vi "水样测试.vi"(11 "数据标记表":string(combo)="N") -> ()   [LabVIEW 2016, in "斯坦道多参数.lvlib"]
panel:
  out "运行状态":u16(ring) items=["空闲", "水样测试", "标样核查"]
  out "多参数运行日志":string
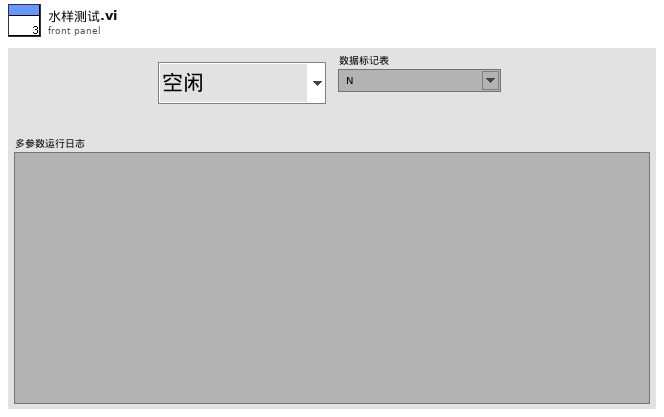
[diagram p1: front panel]
types:
  T1 = cluster{"因子编码":string, "单位":string, "标样参考值":sgl, "水样数据时间":timestamp, "水样实测值":sgl, "水样数据标识":string, "探头温度":sgl}
  T2 = cluster{"温度测量值":sgl, "DO%":sgl, "DOmg/L":sgl, "温度偏移修正值":sgl}
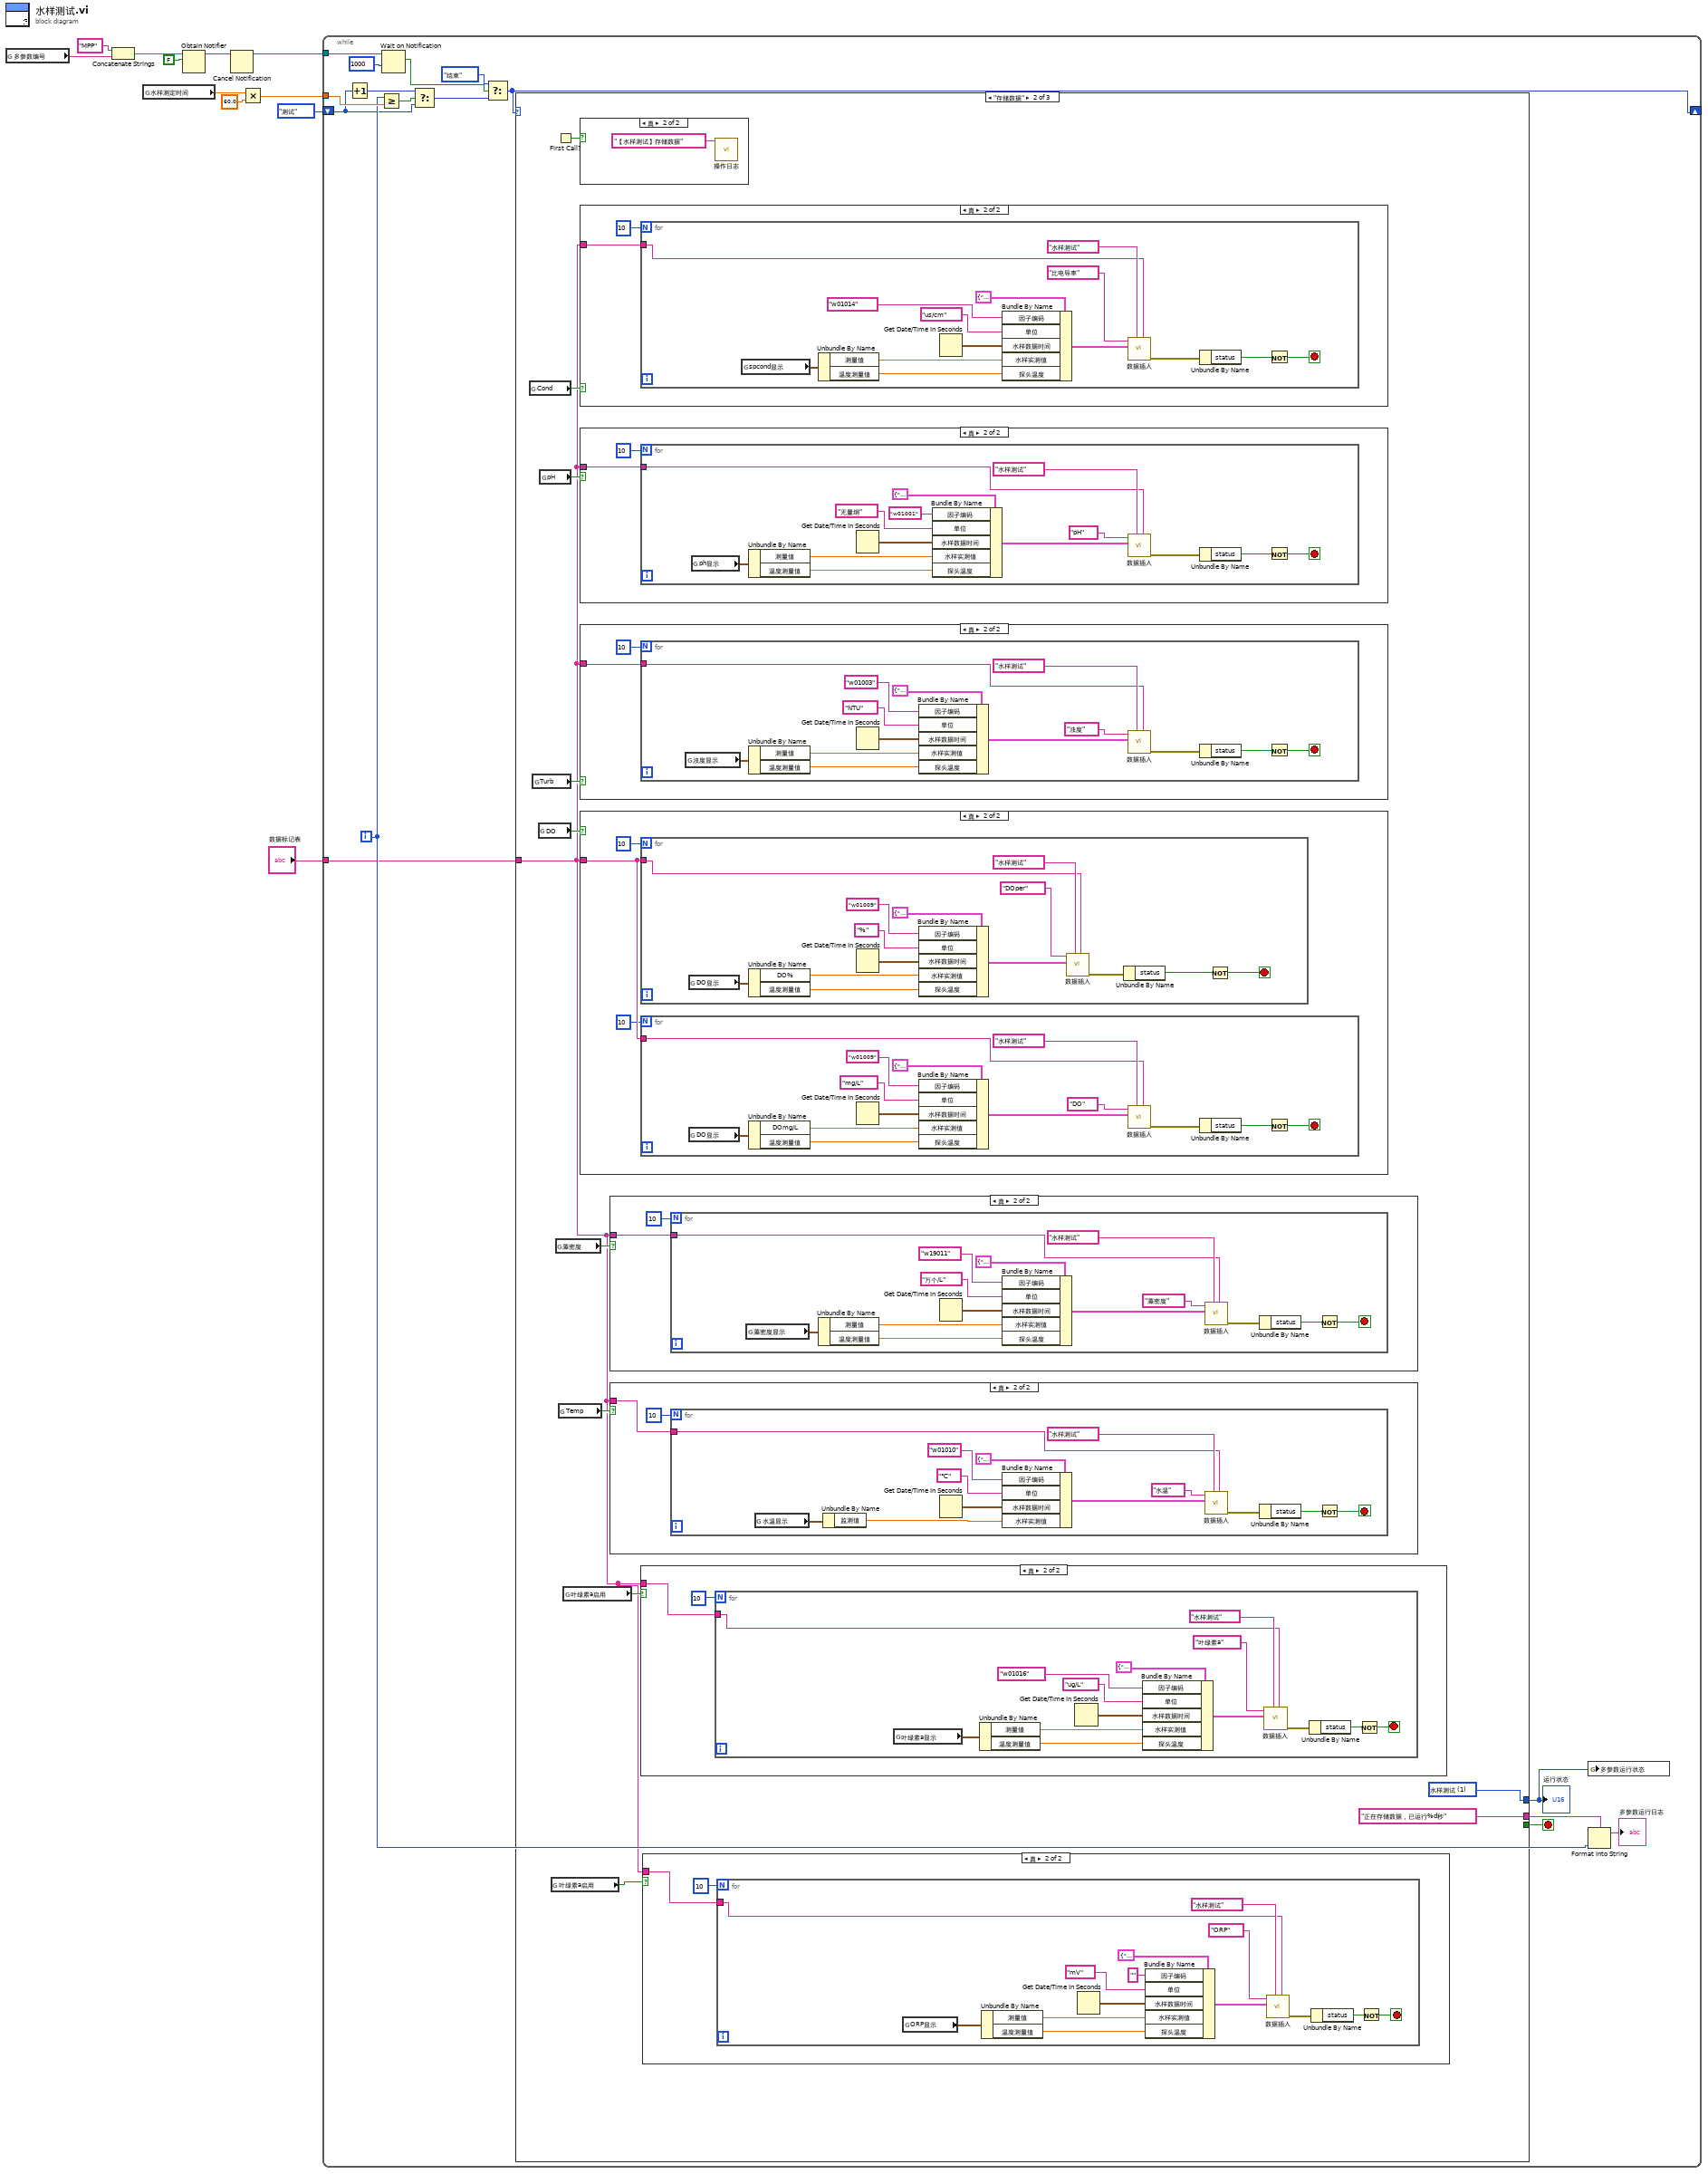
[diagram p0: block diagram]
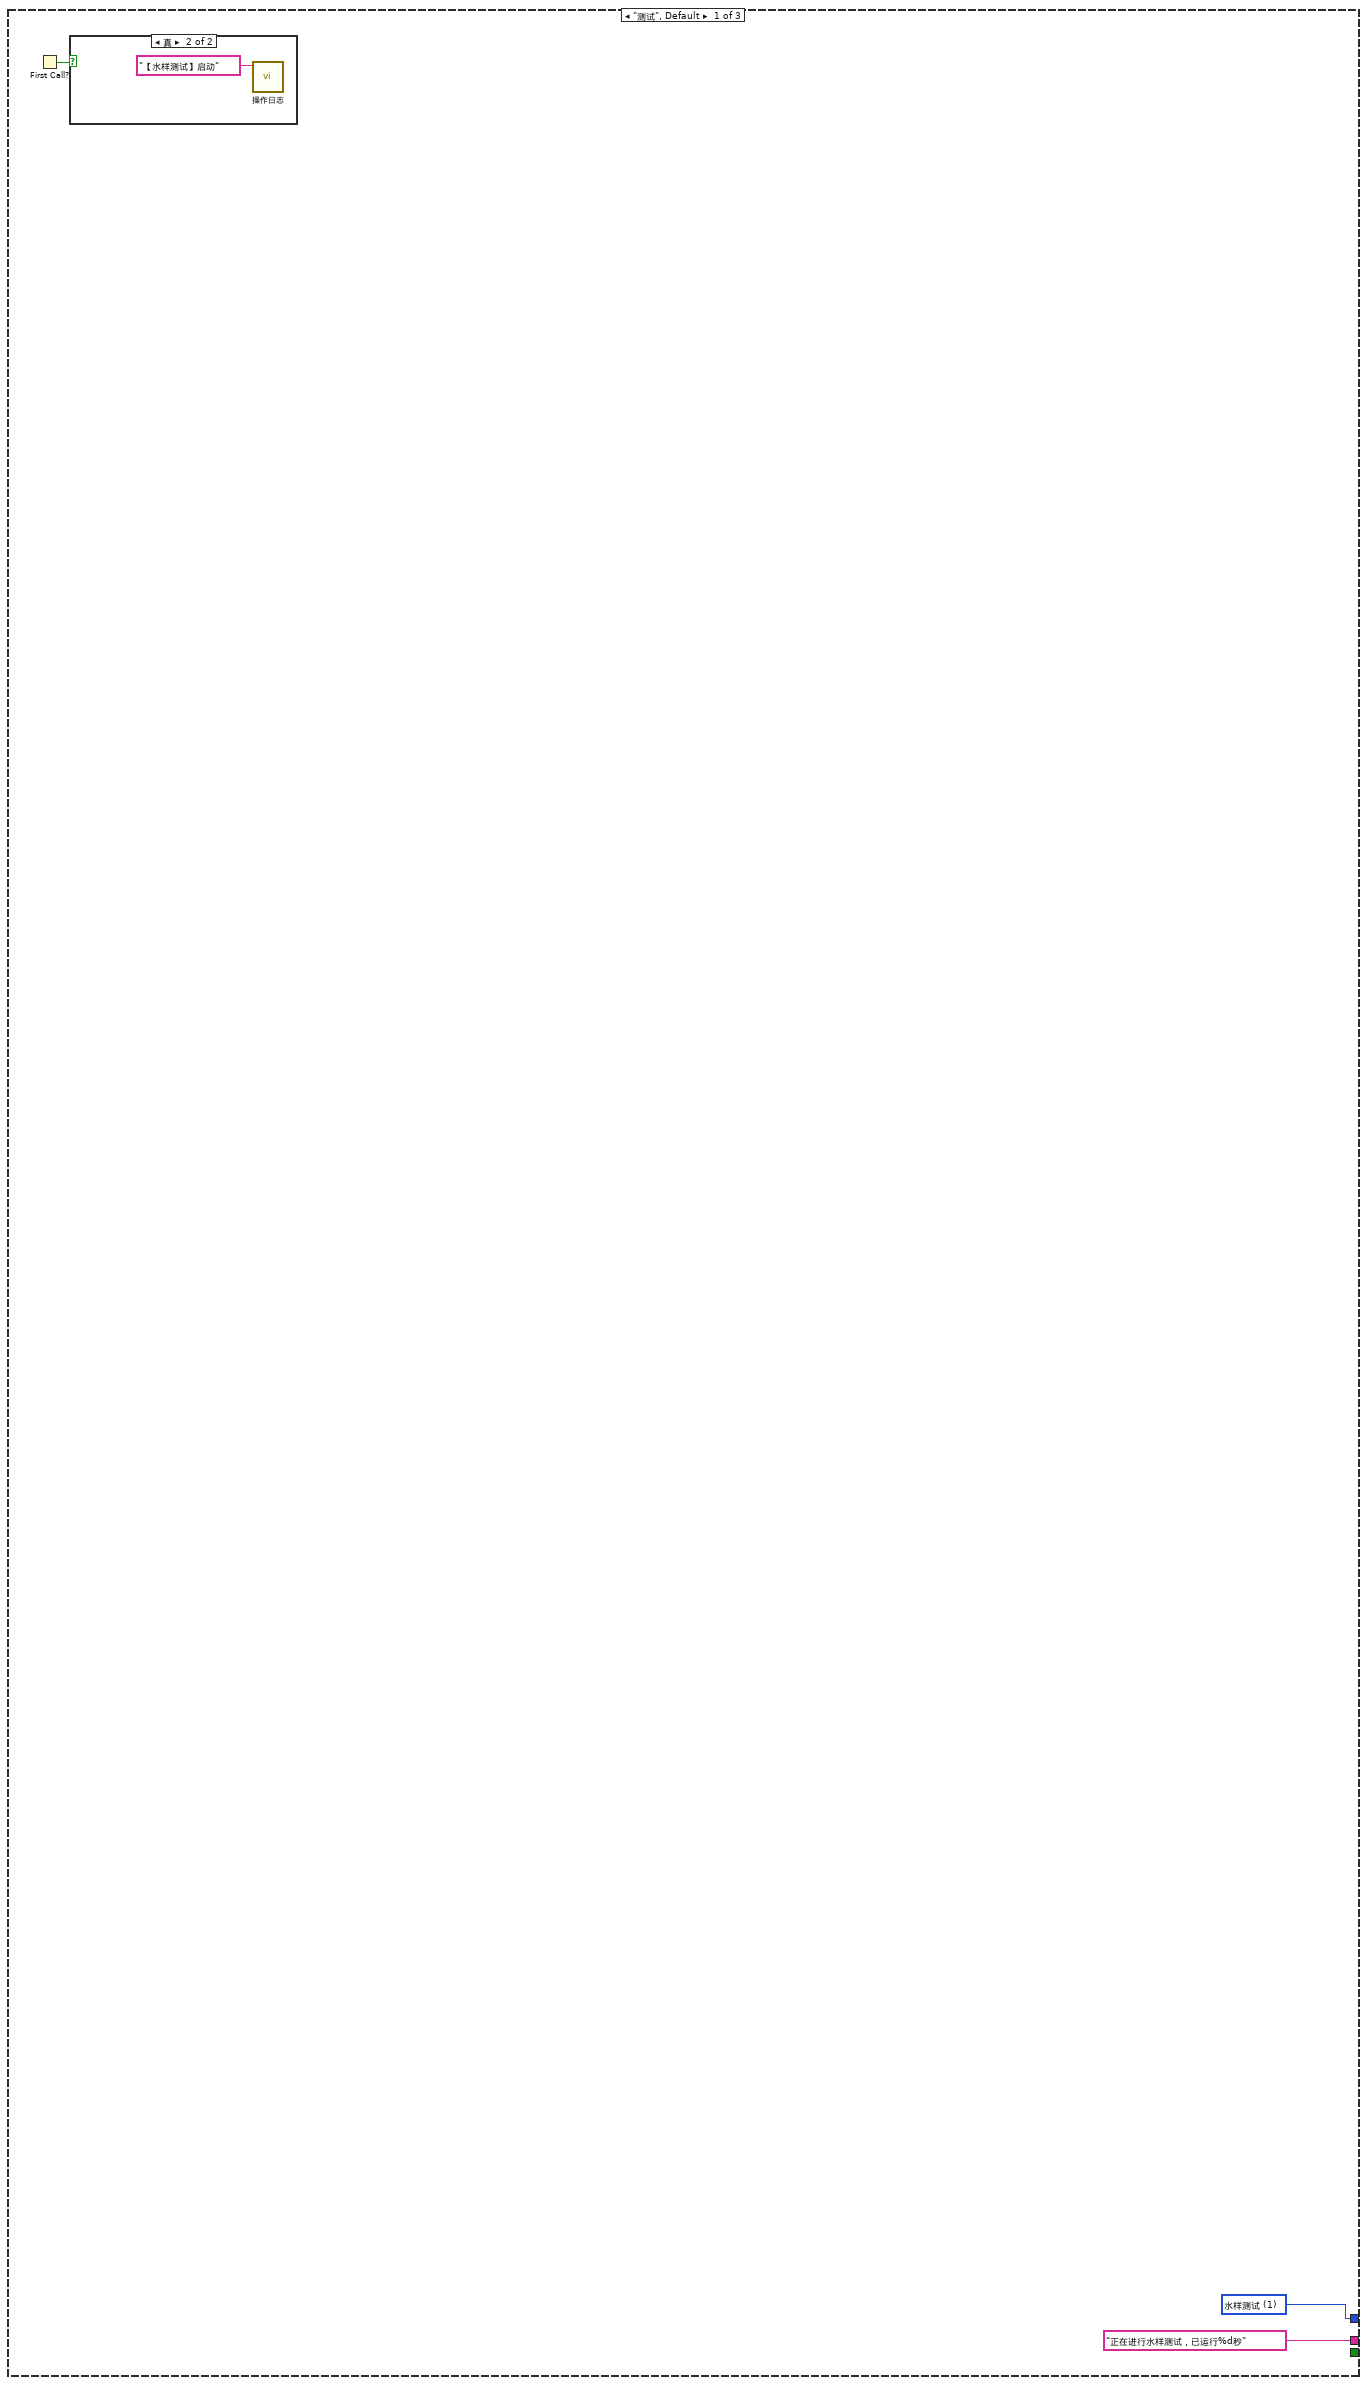
[diagram p2: hidden frame]
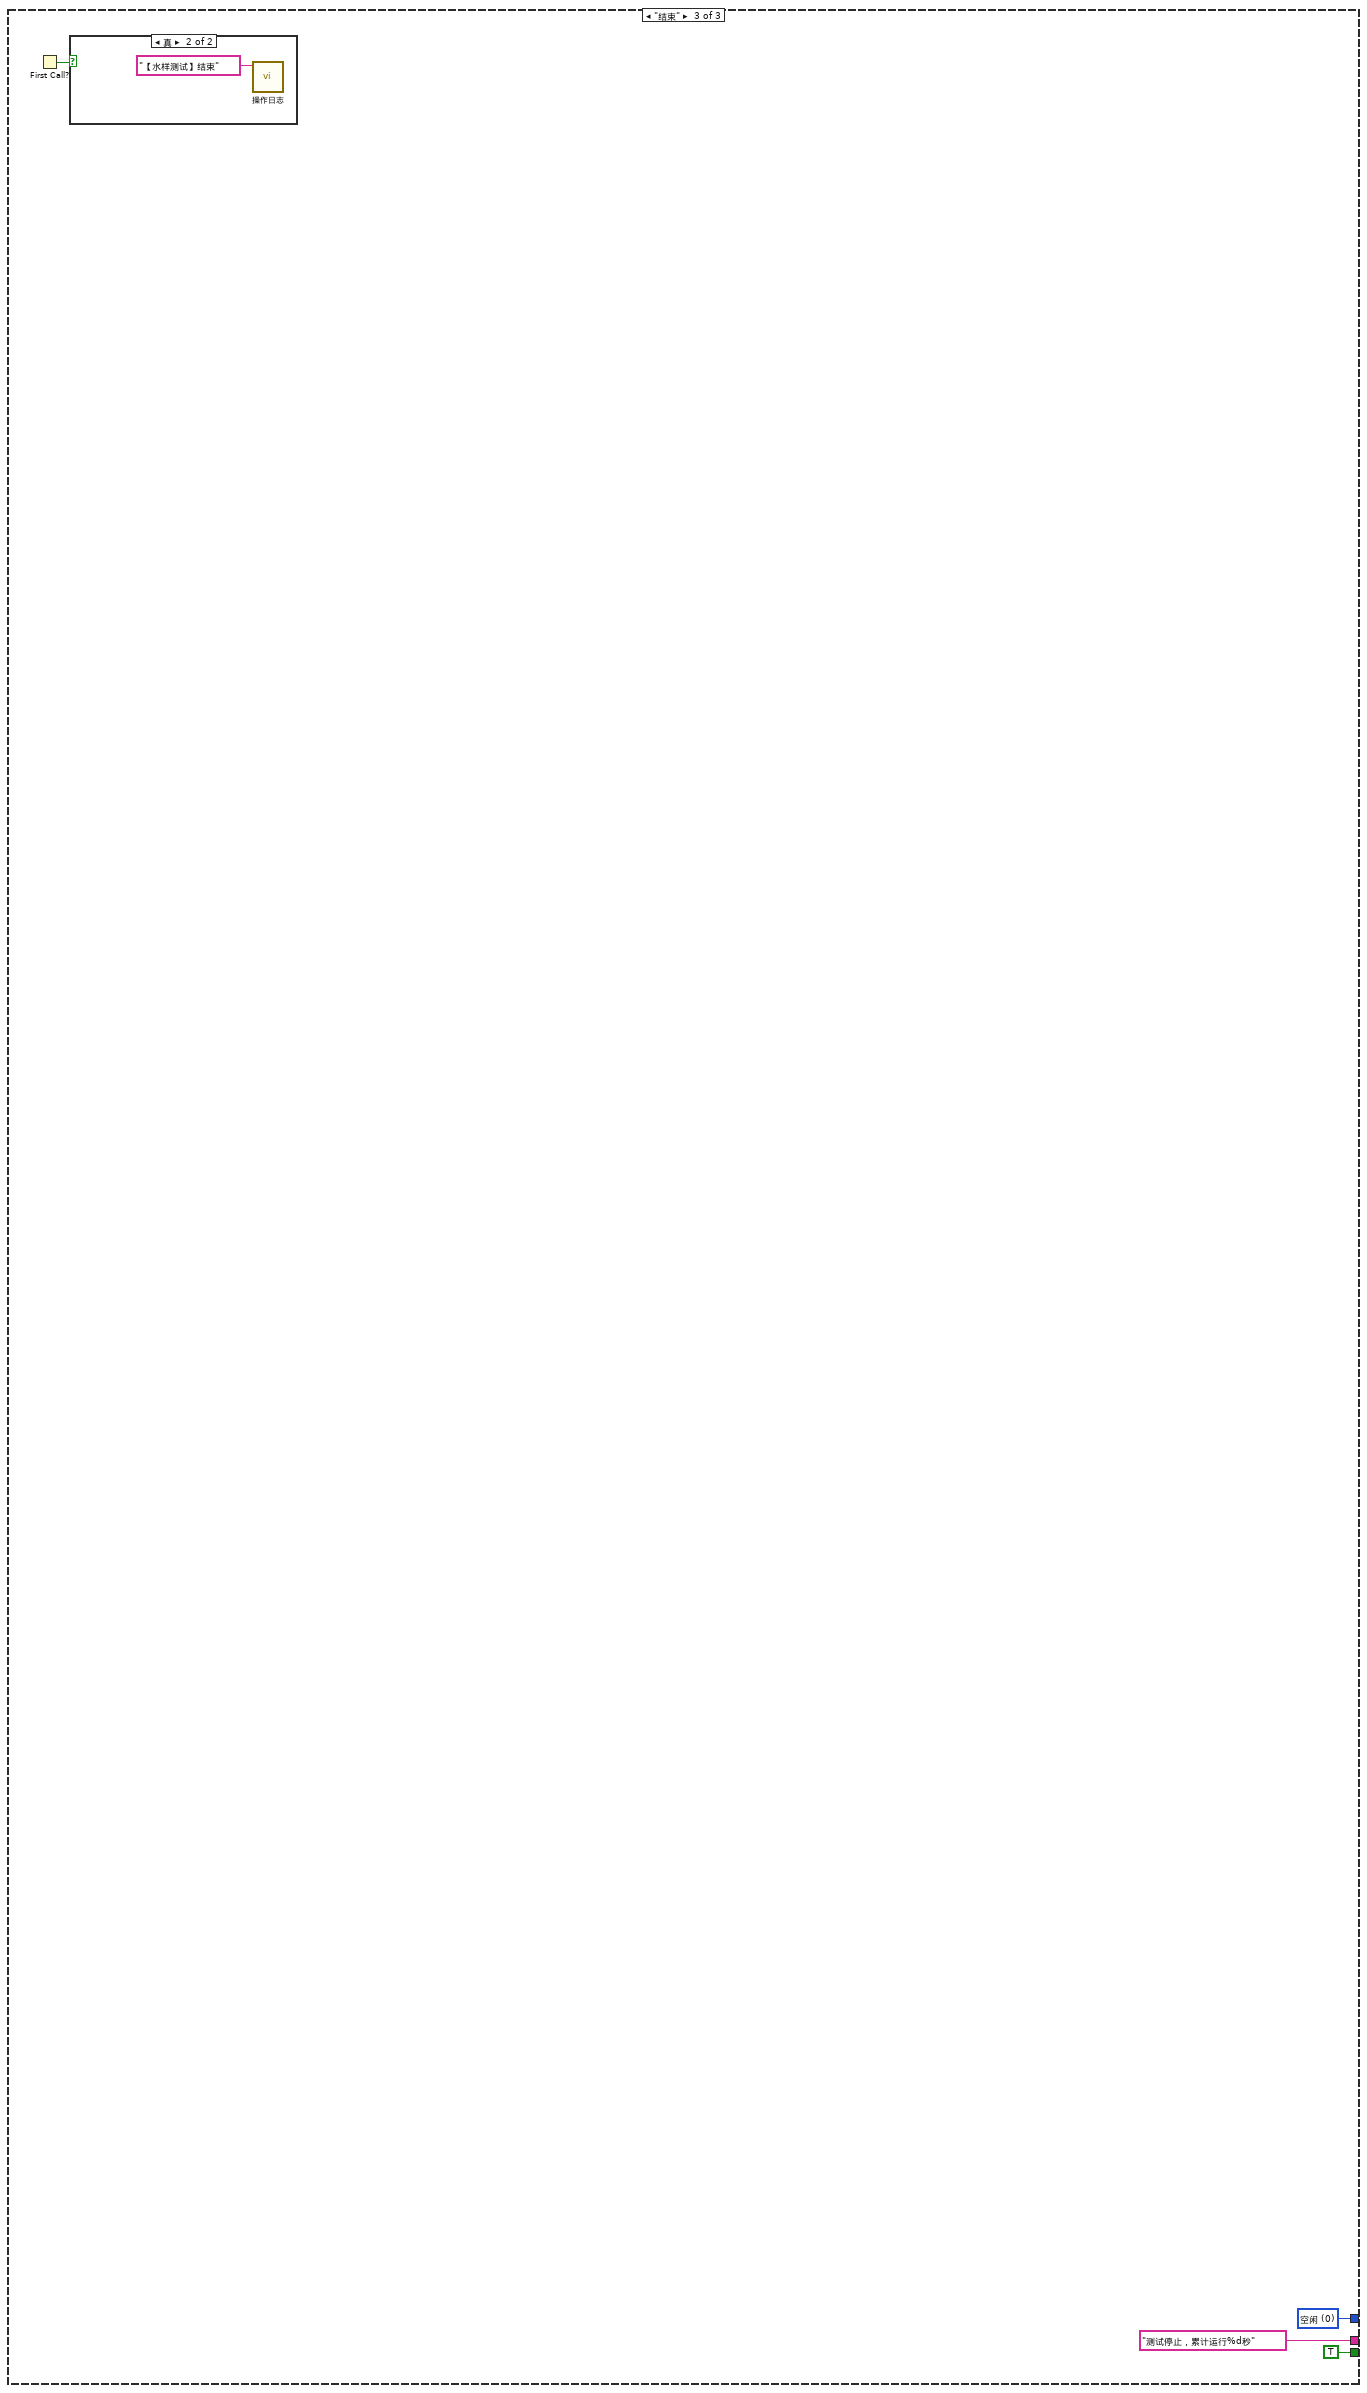
[diagram p13: hidden frame]
diagram:
  n1 = global read "多参数全局变量.vi" "多参数编号"() -> (w2:string)
  n2 = Concatenate Strings("MPP" ("名称（未命名）"), w2) -> (w3:string)
  n3 = global read "断电保存变量.vi" "水样测定时间"() -> (w1:dbl)
  n4 = Obtain Notifier(name (unnamed)=w3, notification data type=FALSE) -> (notifier out=w6:refnum<notifier>)  [unwired: 2 in, 2 out]
  n5 = Cancel Notification(0:w6) -> (8:w5:refnum<notifier>)  [unwired: 1 in, 2 out]
  n6 = Multiply(x=w1, y=60.0) -> (x*y=w10:dbl)
  n7 = while {
    tunnel: w10 -> [w27]
    shift-right: [w14] -> _
    shift-left: enum16{"测试", "存储数据", "结束"}."测试" ("枚举") -> [w21]
    tunnel: w5 -> [w19]
    tunnel: "数据标记表" -> [w13]
    i -> [w25]
    stop <- w26 stop-if-true
    n8 = Increment(x=w21) -> (x+1=w20:enum16{"测试", "存储数据", "结束"})
    n9 = Greater Or Equal?(x=w25, y=w27) -> (x >= y?=w22:bool)
    n10 = Wait on Notification(notifier=w19, timeout in ms (-1)=1000 ("超时毫秒(-1)")) -> (notification=w17:bool)  [unwired: 2 in, 3 out]
    n11 = Select(t=w20, s=w22, f=w21) -> (s? t:f=w15:enum16{"测试", "存储数据", "结束"})
    n12 = Select(t=enum16{"测试", "存储数据", "结束"}."结束" ("枚举"), s=w17, f=w15) -> (s? t:f=w14:enum16{"测试", "存储数据", "结束"})
    n13 = case shown="\"存储数据\"" w14 {
      tunnel: [_ _ TRUE] -> w26
      tunnel: ["正在进行水样测试，已运行%d秒" ("格式字符串") "正在存储数据，已运行%d秒" ("格式字符串") "测试停止，累计运行%d秒" ("格式字符串")] -> w24
      tunnel: [w29 w36 w188] -> w12
      tunnel: w13 -> [_ w33 _]
      frame "测试", Default {
        w29 = u16 1 items=["空闲", "水样测试", "标样核查"] ("多参数运行状态")
        n14 = First Call?() -> (First Call?: T/F=w28:bool)
        n15 = case shown="真" w28 {
          frame False {
          }
          frame True {
            n16 = call "操作日志.vi"("日志信息"="【水样测试】启动") -> ()  [unwired: 10 in, 1 out]
          }
        }
      }
      frame "存储数据" {
        w36 = u16 1 items=["空闲", "水样测试", "标样核查"] ("多参数运行状态")
        n17 = global read "断电保存变量.vi" "Cond"() -> (w41:bool)
        n18 = global read "断电保存变量.vi" "Turb"() -> (w42:bool)
        n19 = global read "断电保存变量.vi" "DO"() -> (w40:bool)
        n20 = global read "断电保存变量.vi" "pH"() -> (w39:bool)
        n21 = global read "断电保存变量.vi" "叶绿素a启用"() -> (w32:bool)
        n22 = First Call?() -> (First Call?: T/F=w34:bool)
        n23 = global read "断电保存变量.vi" "藻密度"() -> (w35:bool)
        n24 = global read "断电保存变量.vi" "Temp"() -> (w38:bool)
        n25 = global read "断电保存变量.vi" "叶绿素a启用"() -> (w43:bool)
        n26 = case shown="真" w34 {
          frame False {
          }
          frame True {
            n27 = call "操作日志.vi"("日志信息"="【水样测试】存储数据") -> ()  [unwired: 10 in, 1 out]
          }
        }
        n28 = case shown="真" w41 {
          tunnel: w33 -> [_ w110]
          frame False {
          }
          frame True {
            n29 = for {
              N: 10 -> [_]
              tunnel: w110 -> [w117]
              stop <- w111 stop-if-true
              n30 = global read "多参数全局变量.vi" "spcond显示"() -> (w116:cluster{"温度测量值":sgl, "测量值":sgl, "温度偏移修正值":sgl})
              n31 = Unbundle By Name(w116) -> ("测量值"=w115:sgl, "温度测量值"=w114:sgl)
              n32 = Get Date/Time In Seconds() -> (seconds since 1Jan1904=w122:timestamp)
              n33 = Bundle By Name(cluster=T1 {"因子编码"="w01003", "单位"="无量纲", "标样参考值"=0.0, "水样数据时间"=timestamp(0 s since 1904-01-01), "水样实测值"=0.0, "水样数据标识"="N", "探头温度"=0.0} ("data in"), "因子编码"="w01014", "单位"="us/cm", "水样数据时间"=w122, "水样实测值"=w115, "探头温度"=w114) -> (w123:T1)
              n34 = call "数据插入.vi"("数据标记表"=w117, "测量模式"="水样测试", "data in"=w123, "table输入"="比电导率") -> ("error out"=w113:errorcluster)  [unwired: 7 in]
              n35 = Unbundle By Name(w113) -> ("status"=w112:bool)
              n36 = Not(x=w112) -> (.not. x?=w111:bool)
            }
          }
        }
        n37 = case shown="真" w39 {
          tunnel: w33 -> [_ w157]
          frame False {
          }
          frame True {
            n38 = for {
              N: 10 -> [_]
              tunnel: w157 -> [w164]
              stop <- w158 stop-if-true
              n39 = global read "多参数全局变量.vi" "ph显示"() -> (w163:cluster{"温度测量值":sgl, "测量值":sgl, "温度偏移修正值":sgl})
              n40 = Unbundle By Name(w163) -> ("测量值"=w162:sgl, "温度测量值"=w161:sgl)
              n41 = Get Date/Time In Seconds() -> (seconds since 1Jan1904=w169:timestamp)
              n42 = Bundle By Name(cluster=T1 {"因子编码"="w01003", "单位"="无量纲", "标样参考值"=0.0, "水样数据时间"=timestamp(0 s since 1904-01-01), "水样实测值"=0.0, "水样数据标识"="N", "探头温度"=0.0} ("data in"), "因子编码"="w01001", "单位"="无量纲", "水样数据时间"=w169, "水样实测值"=w162, "探头温度"=w161) -> (w170:T1)
              n43 = call "数据插入.vi"("数据标记表"=w164, "测量模式"="水样测试", "data in"=w170, "table输入"="pH") -> ("error out"=w160:errorcluster)  [unwired: 7 in]
              n44 = Unbundle By Name(w160) -> ("status"=w159:bool)
              n45 = Not(x=w159) -> (.not. x?=w158:bool)
            }
          }
        }
        n46 = case shown="真" w42 {
          tunnel: w33 -> [_ w94]
          frame False {
          }
          frame True {
            n47 = for {
              N: 10 -> [_]
              tunnel: w94 -> [w101]
              stop <- w95 stop-if-true
              n48 = global read "多参数全局变量.vi" "浊度显示"() -> (w100:cluster{"温度测量值":sgl, "测量值":sgl, "温度偏移修正值":sgl})
              n49 = Unbundle By Name(w100) -> ("测量值"=w99:sgl, "温度测量值"=w98:sgl)
              n50 = Get Date/Time In Seconds() -> (seconds since 1Jan1904=w107:timestamp)
              n51 = Bundle By Name(cluster=T1 {"因子编码"="w01003", "单位"="无量纲", "标样参考值"=0.0, "水样数据时间"=timestamp(0 s since 1904-01-01), "水样实测值"=0.0, "水样数据标识"="N", "探头温度"=0.0} ("data in"), "因子编码"="w01003", "单位"="NTU", "水样数据时间"=w107, "水样实测值"=w99, "探头温度"=w98) -> (w106:T1)
              n52 = call "数据插入.vi"("数据标记表"=w101, "测量模式"="水样测试", "data in"=w106, "table输入"="浊度") -> ("error out"=w97:errorcluster)  [unwired: 7 in]
              n53 = Unbundle By Name(w97) -> ("status"=w96:bool)
              n54 = Not(x=w96) -> (.not. x?=w95:bool)
            }
          }
        }
        n55 = case shown="真" w40 {
          tunnel: w33 -> [_ w127]
          frame False {
          }
          frame True {
            n56 = for {
              N: 10 -> [_]
              tunnel: w127 -> [w140]
              stop <- w128 stop-if-true
              n57 = global read "多参数全局变量.vi" "DO显示"() -> (w131:T2)
              n58 = Unbundle By Name(w131) -> ("DO%"=w135:sgl, "温度测量值"=w133:sgl)
              n59 = Get Date/Time In Seconds() -> (seconds since 1Jan1904=w136:timestamp)
              n60 = Bundle By Name(cluster=T1 {"因子编码"="w01003", "单位"="无量纲", "标样参考值"=0.0, "水样数据时间"=timestamp(0 s since 1904-01-01), "水样实测值"=0.0, "水样数据标识"="N", "探头温度"=0.0} ("data in"), "因子编码"="w01009", "单位"="%", "水样数据时间"=w136, "水样实测值"=w135, "探头温度"=w133) -> (w132:T1)
              n61 = call "数据插入.vi"("数据标记表"=w140, "测量模式"="水样测试", "data in"=w132, "table输入"="DOper") -> ("error out"=w130:errorcluster)  [unwired: 7 in]
              n62 = Unbundle By Name(w130) -> ("status"=w129:bool)
              n63 = Not(x=w129) -> (.not. x?=w128:bool)
            }
            n64 = for {
              N: 10 -> [_]
              tunnel: w127 -> [w148]
              stop <- w142 stop-if-true
              n65 = global read "多参数全局变量.vi" "DO显示"() -> (w147:T2)
              n66 = Unbundle By Name(w147) -> ("DOmg/L"=w146:sgl, "温度测量值"=w145:sgl)
              n67 = Get Date/Time In Seconds() -> (seconds since 1Jan1904=w154:timestamp)
              n68 = Bundle By Name(cluster=T1 {"因子编码"="w01003", "单位"="无量纲", "标样参考值"=0.0, "水样数据时间"=timestamp(0 s since 1904-01-01), "水样实测值"=0.0, "水样数据标识"="N", "探头温度"=0.0} ("data in"), "因子编码"="w01009", "单位"="mg/L", "水样数据时间"=w154, "水样实测值"=w146, "探头温度"=w145) -> (w153:T1)
              n69 = call "数据插入.vi"("数据标记表"=w148, "测量模式"="水样测试", "data in"=w153, "table输入"="DO") -> ("error out"=w144:errorcluster)  [unwired: 7 in]
              n70 = Unbundle By Name(w144) -> ("status"=w143:bool)
              n71 = Not(x=w143) -> (.not. x?=w142:bool)
            }
          }
        }
        n72 = case shown="真" w35 {
          tunnel: w33 -> [_ w62]
          frame False {
          }
          frame True {
            n73 = for {
              N: 10 -> [_]
              tunnel: w62 -> [w67]
              stop <- w63 stop-if-true
              n74 = global read "多参数全局变量.vi" "藻密度显示"() -> (w66:cluster{"温度测量值":sgl, "测量值":sgl, "温度偏移修正值":sgl})
              n75 = Unbundle By Name(w66) -> ("测量值"=w74:sgl, "温度测量值"=w72:sgl)
              n76 = Get Date/Time In Seconds() -> (seconds since 1Jan1904=w75:timestamp)
              n77 = Bundle By Name(cluster=T1 {"因子编码"="w01003", "单位"="无量纲", "标样参考值"=0.0, "水样数据时间"=timestamp(0 s since 1904-01-01), "水样实测值"=0.0, "水样数据标识"="N", "探头温度"=0.0} ("data in"), "因子编码"="w19011", "单位"="万个/L", "水样数据时间"=w75, "水样实测值"=w74, "探头温度"=w72) -> (w70:T1)
              n78 = call "数据插入.vi"("数据标记表"=w67, "测量模式"="水样测试", "data in"=w70, "table输入"="藻密度") -> ("error out"=w65:errorcluster)  [unwired: 7 in]
              n79 = Unbundle By Name(w65) -> ("status"=w64:bool)
              n80 = Not(x=w64) -> (.not. x?=w63:bool)
            }
          }
        }
        n81 = case shown="真" w38 {
          tunnel: w33 -> [_ w173]
          frame False {
          }
          frame True {
            n82 = for {
              N: 10 -> [_]
              tunnel: w173 -> [w179]
              stop <- w174 stop-if-true
              n83 = global read "多参数全局变量.vi" "水温显示"() -> (w178:cluster{"CH":u16, "监测值":dbl, "温度偏移修正值":sgl})
              n84 = Unbundle By Name(w178) -> ("监测值"=w177:dbl)
              n85 = Get Date/Time In Seconds() -> (seconds since 1Jan1904=w185:timestamp)
              n86 = Bundle By Name(cluster=T1 {"因子编码"="w01003", "单位"="无量纲", "标样参考值"=0.0, "水样数据时间"=timestamp(0 s since 1904-01-01), "水样实测值"=0.0, "水样数据标识"="N", "探头温度"=0.0} ("data in"), "因子编码"="w01010", "单位"="℃", "水样数据时间"=w185, "水样实测值"=w177) -> (w184:T1)
              n87 = call "数据插入.vi"("数据标记表"=w179, "测量模式"="水样测试", "data in"=w184, "table输入"="水温") -> ("error out"=w176:errorcluster)  [unwired: 7 in]
              n88 = Unbundle By Name(w176) -> ("status"=w175:bool)
              n89 = Not(x=w175) -> (.not. x?=w174:bool)
            }
          }
        }
        n90 = case shown="真" w43 {
          tunnel: w33 -> [_ w78]
          frame False {
          }
          frame True {
            n91 = for {
              N: 10 -> [_]
              tunnel: w78 -> [w83]
              stop <- w79 stop-if-true
              n92 = global read "多参数全局变量.vi" "叶绿素a显示"() -> (w82:cluster{"温度测量值":sgl, "测量值":sgl, "温度偏移修正值":sgl})
              n93 = Unbundle By Name(w82) -> ("测量值"=w90:sgl, "温度测量值"=w88:sgl)
              n94 = Get Date/Time In Seconds() -> (seconds since 1Jan1904=w91:timestamp)
              n95 = Bundle By Name(cluster=T1 {"因子编码"="w01003", "单位"="无量纲", "标样参考值"=0.0, "水样数据时间"=timestamp(0 s since 1904-01-01), "水样实测值"=0.0, "水样数据标识"="N", "探头温度"=0.0} ("data in"), "因子编码"="w01016", "单位"="ug/L", "水样数据时间"=w91, "水样实测值"=w90, "探头温度"=w88) -> (w86:T1)
              n96 = call "数据插入.vi"("数据标记表"=w83, "测量模式"="水样测试", "data in"=w86, "table输入"="叶绿素a") -> ("error out"=w81:errorcluster)  [unwired: 7 in]
              n97 = Unbundle By Name(w81) -> ("status"=w80:bool)
              n98 = Not(x=w80) -> (.not. x?=w79:bool)
            }
          }
        }
        n99 = case shown="真" w32 {
          tunnel: w33 -> [_ w45]
          frame False {
          }
          frame True {
            n100 = for {
              N: 10 -> [_]
              tunnel: w45 -> [w51]
              stop <- w47 stop-if-true
              n101 = global read "多参数全局变量.vi" "ORP显示"() -> (w50:cluster{"温度测量值":sgl, "测量值":sgl, "温度偏移修正值":sgl})
              n102 = Unbundle By Name(w50) -> ("测量值"=w57:sgl, "温度测量值"=w55:sgl)
              n103 = Get Date/Time In Seconds() -> (seconds since 1Jan1904=w58:timestamp)
              n104 = Bundle By Name(cluster=T1 {"因子编码"="w01003", "单位"="无量纲", "标样参考值"=0.0, "水样数据时间"=timestamp(0 s since 1904-01-01), "水样实测值"=0.0, "水样数据标识"="N", "探头温度"=0.0} ("data in"), "因子编码"="", "单位"="mV", "水样数据时间"=w58, "水样实测值"=w57, "探头温度"=w55) -> (w53:T1)
              n105 = call "数据插入.vi"("数据标记表"=w51, "测量模式"="水样测试", "data in"=w53, "table输入"="ORP") -> ("error out"=w49:errorcluster)  [unwired: 7 in]
              n106 = Unbundle By Name(w49) -> ("status"=w48:bool)
              n107 = Not(x=w48) -> (.not. x?=w47:bool)
            }
          }
        }
      }
      frame "结束" {
        w188 = u16 0 items=["空闲", "水样测试", "标样核查"] ("多参数运行状态")
        n108 = First Call?() -> (First Call?: T/F=w187:bool)
        n109 = case shown="真" w187 {
          frame False {
          }
          frame True {
            n110 = call "操作日志.vi"("日志信息"="【水样测试】结束") -> ()  [unwired: 10 in, 1 out]
          }
        }
      }
    }
    "运行状态" <- w12
    n111 = global write "多参数全局变量.vi" "多参数运行状态"(w12) -> ()
    n112 = Format Into String(format string=w24, w25) -> (resulting string=→"多参数运行日志":string)  [unwired: 2 in, 1 out]
  }
